vi "Configure Shutdown Timer.vi"(8 "error in (no error)":errorcluster, 9 "Shutdown Timer (0)":i16 min=0 max=1000 step=1, 11 "VISA resource name":refnum<visa-resource-name>) -> (0 "error out":errorcluster, 3 "VISA resource name out":refnum<visa-resource-name>)   [LabVIEW 2012, in "Temptronic TP04300.lvlib"]
doc: "This VI configures a shutdown timer for TP04300 instrument.\n\n<b>Shutdown Timer</b> - used to configure the time in minutes before system shuts down.\n\nDefault Value: 0 - shutdown timer disabled\nValid Range: 0 - 1000"
uses:
  <instrlib>/Temptronic TP04300/Temptronic TP04300.lvlib
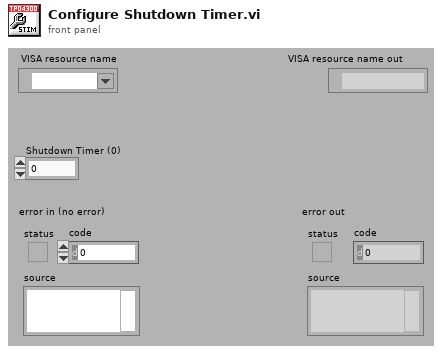
[diagram p1: front panel]
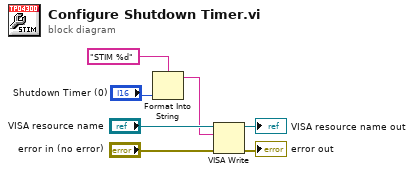
[diagram p0: block diagram]
diagram:
  n1 = Format Into String(format string="STIM %d" ("multi-line string"), "Shutdown Timer (0)") -> (resulting string=w3:string)  [unwired: 2 in, 1 out]
  n2 = VISA Write(VISA resource name="VISA resource name", write buffer=w3, error in (no error)="error in (no error)") -> (VISA resource name out=→"VISA resource name out":refnum<visa-resource-name>, error out=→"error out":errorcluster)  [unwired: 1 out]
